vi "Build Data Package for Host.vi"(9 "Tick Number(U32)":u32, 11 "IO States(U32)":u32) -> (3 "Data to Host (U64)":u64)   [LabVIEW 2016]
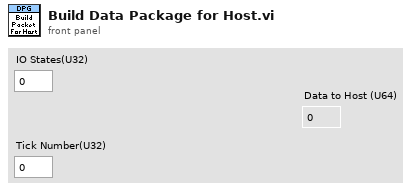
[diagram p1: front panel]
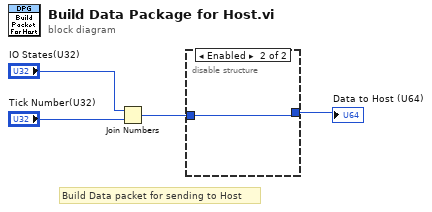
[diagram p0: block diagram]
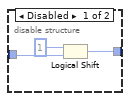
[diagram p2: hidden frame]
diagram:
  # "Build Data packet for sending to Host"
  n1 = Join Numbers(hi="IO States(U32)", lo="Tick Number(U32)") -> ((hi.lo)=w2:u64)
  n2 = disable-structure shown="Enabled" {
    disable-tunnel: w2 -> [w7 w8]
    disable-tunnel: [w6 w8] -> w1
    frame Disabled {
      n3 = Logical Shift(y=i16 1, x=w7) -> (x << y=w6:u64)
    }
    frame Enabled {
    }
  }
  "Data to Host (U64)" <- w1
